vi "Make Screenshots.vi"() -> ()   [LabVIEW 2021]
panel:
  in  "ImageFolder":path
  out "Array 2":string[](array[string])
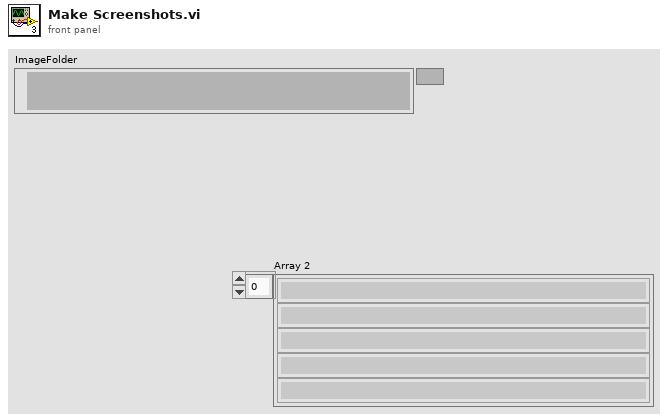
[diagram p1: front panel]
types:
  T1 = typedef "LVBookmarkInfoTypeDef.ctl" = cluster{"Bookmark Reference":u32, "Bookmark Tag":string, "Label Text":string}[]
  T2 = typedef "imagedata.ctl" = cluster{"image type":i32, "image depth":i32, "image":u8[], "mask":u8[], "colors":u32[], "Rectangle":cluster{"left":i16, "top":i16, "right":i16, "bottom":i16}}
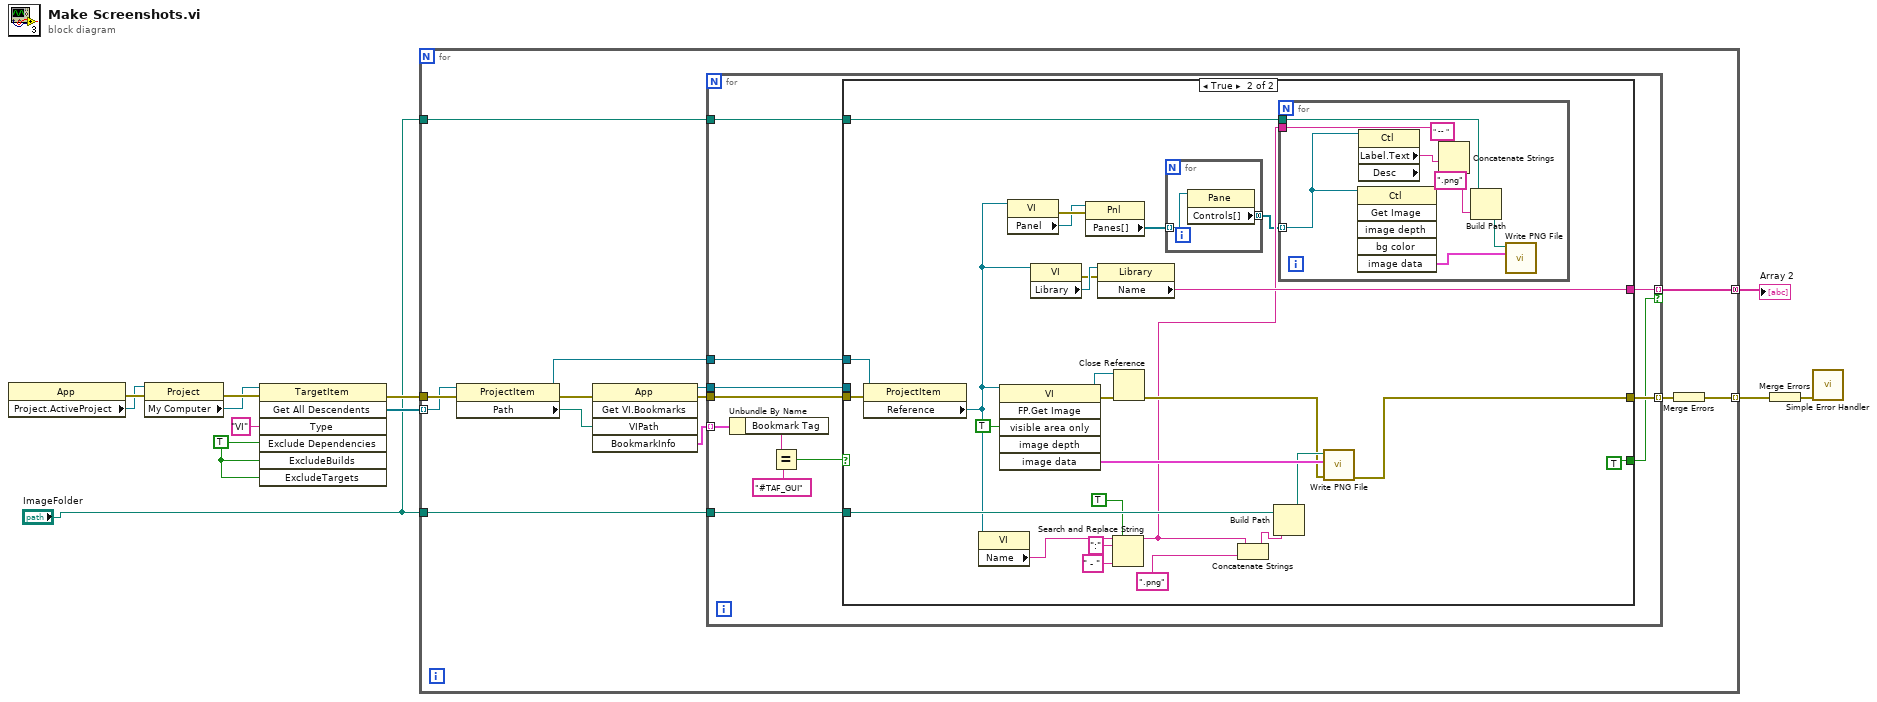
[diagram p0: block diagram]
diagram:
  w7 = TRUE ("ExcludeDependencies")
  n1 = property class="App"() -> (error out=w12:errorcluster, "Project.ActiveProject"=w11:refnum<vi>)  [unwired: 2 in, 1 out]
  n2 = property class="Project"(reference=w11, error in=w12) -> (error out=w10:errorcluster, "My Computer"=w9:refnum<vi>)  [unwired: 1 out]
  n3 = invoke class="TargetItem" method="Get All Descendents"(reference=w9, error in=w10, "Type"="VI", "Exclude Dependencies"=w7, "ExcludeBuilds"=w7, "ExcludeTargets"=w7) -> (error out=w5:errorcluster, "All Descendents"=w6:refnum<vi>[])  [unwired: 1 in, 5 out]
  n4 = for {
    tunnel: w6 -> [w24] mode=indexing
    tunnel: w5 -> [w25]
    tunnel: [w21] -> w4 mode=indexing
    tunnel: [w20] -> w2 mode=concatenating
    tunnel: "ImageFolder" -> [w19]
    tunnel: "ImageFolder" -> [w18]
    n5 = property class="ProjectItem"(reference=w24, error in=w25) -> (reference out=w16:refnum<vi>, error out=w13:errorcluster, "Path"=w14:path)
    n6 = invoke class="App" method="Get VI.Bookmarks"(error in=w13, "VIPath"=w14) -> (reference out=w17:refnum<vi>, error out=w23:errorcluster, "BookmarkInfo"=w15:T1)  [unwired: 3 in, 2 out]
    n7 = for {
      tunnel: w15 -> [w37] mode=indexing
      tunnel: w23 -> [w27]
      tunnel: [w33] -> w22 mode=indexing
      tunnel: [w32] -> w20 mode=indexing if=w31
      tunnel: w19 -> [w30]
      tunnel: w18 -> [w29]
      tunnel: w17 -> [w28]
      tunnel: w16 -> [w26]
      n8 = Unbundle By Name(w37) -> ("Bookmark Tag"=w36:string)
      n9 = Equal?(x=w36, y="#TAF_GUI") -> (x = y?=w34:bool)
      n10 = case shown="True" w34 {
        tunnel: [_ TRUE] -> w31
        tunnel: [w38 w56] -> w33
        tunnel: [_ w61] -> w32
        tunnel: w30 -> [_ w59]
        tunnel: w29 -> [_ w49]
        tunnel: w28 -> [_ _]
        tunnel: w27 -> [w38 w41]
        tunnel: w26 -> [_ w40]
        frame False {
        }
        frame True {
          n11 = property class="ProjectItem"(reference=w40, error in=w41) -> ("Reference"=w39:refnum<vi>)  [unwired: 2 out]
          n12 = property class="VI"(reference=w39) -> ("Name"=w48:string)  [unwired: 1 in, 2 out]
          n13 = invoke class="VI" method="FP.Get Image"(reference=w39, "visible area only"=TRUE ("Visible Area Only")) -> (reference out=w63:refnum<vi>, error out=w64:errorcluster, "image data"=w60:T2)  [unwired: 4 in, 3 out]
          n14 = property class="VI"(reference=w39) -> (error out=w51:errorcluster, "Panel"=w44:refnum<vi>)  [unwired: 1 in, 1 out]
          n15 = property class="VI"(reference=w39) -> (error out=w50:errorcluster, "Library"=w52:refnum<vi>)  [unwired: 1 in, 1 out]
          n16 = property class="Pnl"(reference=w44, error in=w51) -> ("Panes[]"=w43:refnum<vi>[])  [unwired: 2 out]
          n17 = property class="Library"(reference=w52, error in=w50) -> ("Name"=w61:string)  [unwired: 2 out]
          n18 = Search and Replace String(replace all?=TRUE ("replace all? (F)"), input string=w48, search string=":", replace string=" - " ("replace string (\"\")")) -> (result string=w45:string)  [unwired: 4 in, 3 out]
          n19 = Close Reference(reference=w63, error in (no error)=w64) -> (error out=w57:errorcluster)
          n20 = for {
            tunnel: w43 -> [w67] mode=indexing
            tunnel: [w66] -> w42 mode=concatenating
            n21 = property class="Pane"(reference=w67) -> ("Controls[]"=w66:refnum<vi>[])  [unwired: 1 in, 2 out]
          }
          n22 = Concatenate Strings(w45, ".png" ("string")) -> (w47:string)
          n23 = Build Path(base path=w59, name or relative path=w47) -> (appended path=w58:path)
          n24 = for {
            tunnel: w42 -> [w76] mode=indexing
            tunnel: w49 -> [w74]
            tunnel: w45 -> [w73]
            n25 = invoke class="Ctl" method="Get Image"(reference=w76) -> ("image data"=w75:T2)  [unwired: 5 in, 5 out]
            n26 = property class="Ctl" props=["Label", "Text", "Desc"](reference=w76) -> ("Label.Text"=w72:string)  [unwired: 1 in, 3 out]
            n27 = Concatenate Strings(w73, " -- " ("string"), w72, ".png" ("string")) -> (w69:string)
            n28 = Build Path(base path=w74, name or relative path=w69) -> (appended path=w68:path)
            n29 = call <vilib>:"Write PNG File.vi"("image data"=w75, "path to PNG file"=w68) -> ()  [unwired: 8 in, 2 out]
          }
          n30 = call <vilib>:"Write PNG File.vi"("error in (no error)"=w57, "image data"=w60, "path to PNG file"=w58) -> ("error out"=w56:errorcluster)  [unwired: 7 in, 1 out]
        }
      }
    }
    n31 = Merge Errors(w22) -> (w21:errorcluster)
  }
  "Array 2" <- w2
  n32 = Merge Errors(w4) -> (w3:errorcluster)
  n33 = call <vilib>:"Simple Error Handler.vi"("error in (no error)"=w3) -> ()  [unwired: 4 in, 5 out]
